vi "Compra Realizada.vi"(8 "error in (no error)":errorcluster, 10 "producto y costo Cluster":T1) -> (0 "error out":errorcluster)   [LabVIEW 2020, in "Mensajes.lvlib"]
doc: "Se realizo la compra de un producto del inventario\n_____\nCreated using Delacor QMH Event Scripter 5.0.0.112."
uses:
  Mensajes.lvlib
  Compra Realizada Argument--cluster.ctl
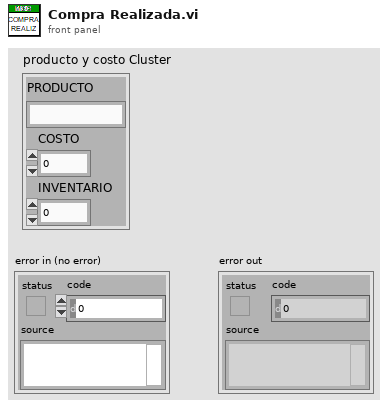
[diagram p1: front panel]
types:
  T1 = cluster{"PRODUCTO":string, "COSTO":dbl, "INVENTARIO":dbl}
  T2 = typedef "Mensajes.lvlib/Compra Realizada Argument--cluster.ctl" = cluster{"producto y costo Cluster":cluster{"PRODUCTO":string, "COSTO":dbl, "INVENTARIO":dbl}}
  T3 = typedef "Mensajes.lvlib/Request Events--cluster.ctl" = cluster{"Stop Module":refnum<user-event>, "Show Panel":refnum<user-event>, "Hide Panel":refnum<user-event>, "Get Module Execution Status":refnum<user-event>, "Show Diagram":refnum<user-event>, "Publicar mensaje":refnum<user-event>, "actualizar el credito":refnum<user-event>, "Compra Realizada":refnum<user-event>}
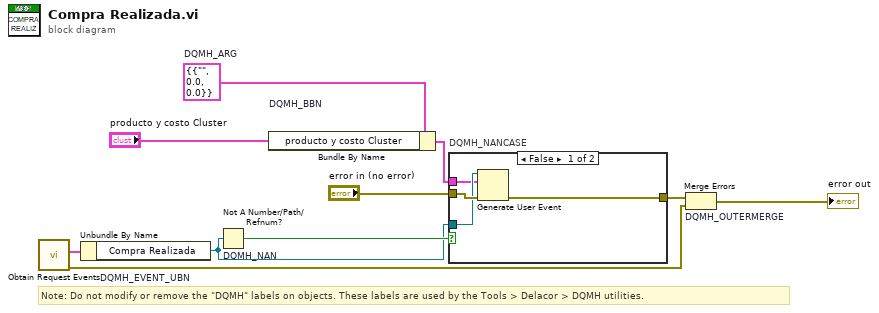
[diagram p0: block diagram]
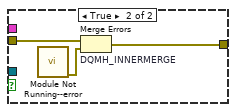
[diagram p2: hidden frame]
diagram:
  w4 = T2 {"producto y costo Cluster"={"PRODUCTO"="", "COSTO"=0.0, "INVENTARIO"=0.0}}  # DQMH_ARG
  # "Note: Do not modify or remove the \"DQMH\" labels on objects. These labels are used by the Tools > Delacor > DQMH utilities."
  n1 = call "Obtain Request Events.vi"() -> ("error out"=w2:errorcluster, "Mensajes Request Events"=w1:T3)  [unwired: 10 in]
  n2 = Unbundle By Name "DQMH_EVENT_UBN"(w1) -> ("Compra Realizada"=w6:refnum<user-event>)
  n3 = Not A Number/Path/Refnum? "DQMH_NAN"(number/path/refnum=w6) -> (NaN/Path/Refnum?=w7:bool)
  n4 = Bundle By Name "DQMH_BBN"(cluster=w4, "producto y costo Cluster"="producto y costo Cluster") -> (w8:T2)
  n5 = case "DQMH_NANCASE" shown="False" w7 {
    tunnel: "error in (no error)" -> [w14 w17]
    tunnel: [w13 w16] -> w5
    tunnel: w6 -> [w12 _]
    tunnel: w8 -> [w11 _]
    frame False {
      n6 = Generate User Event(user event=w12, event data cluster=w11, error in=w14) -> (error out=w13:errorcluster)  [unwired: 1 in, 1 out]
    }
    frame True {
      n7 = call "Module Not Running--error.vi"() -> ("error out"=w15:errorcluster)  [unwired: 11 in]
      n8 = Merge Errors "DQMH_INNERMERGE"(w17, w15) -> (w16:errorcluster)
    }
  }
  n9 = Merge Errors "DQMH_OUTERMERGE"(w5, w2) -> (→"error out":errorcluster)
